vi "Receive.vi"   [LabVIEW 2013, in "I2S-TDM.lvlib"]
uses:
  I2S-TDM.lvlib
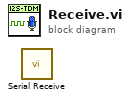
[diagram p0: block diagram]
diagram:
  n1 = call "Serial Receive.vi"() -> ()  [unwired: 10 in, 2 out]
